vi "Fetch Check-out Details.vi"(0 "Central Data Manager in":refnum<class "Central Data Manager.lvclass">, 5 "Rooms Manager GUID":string, 7 "Room No":string, 11 "error in (no error)":errorcluster) -> (4 "Central Data Manager out":refnum<class "Central Data Manager.lvclass">, 15 "error out":errorcluster)   [LabVIEW 2023, in "Central Data Manager.lvlib" / "Central Data Manager.lvclass"]
uses:
  Central Data Manager.lvclass
  Central Data Manager.lvclass/Central Data Manager.ctl
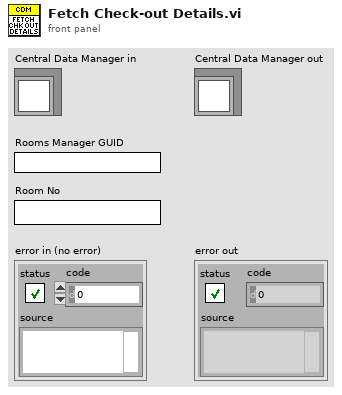
[diagram p1: front panel]
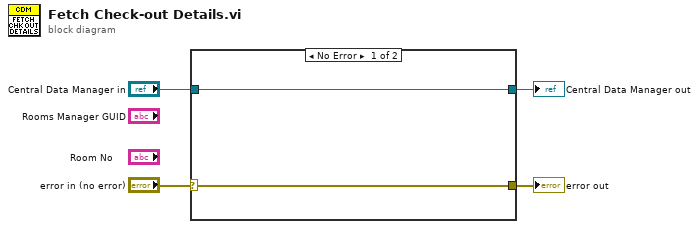
[diagram p0: block diagram]
diagram:
  n1 = case shown="No Error" "error in (no error)" {
    selector: "error in (no error)" -> [w5 w8]
    tunnel: [w5 w8] -> w3
    tunnel: [w6 w7] -> w1
    tunnel: "Central Data Manager in" -> [w6 w7]
    frame No Error {
    }
    frame Error {
    }
  }
  "error out" <- w3
  "Central Data Manager out" <- w1
